vi "Test Bumpy Terrain.vi"   [LabVIEW 2017]
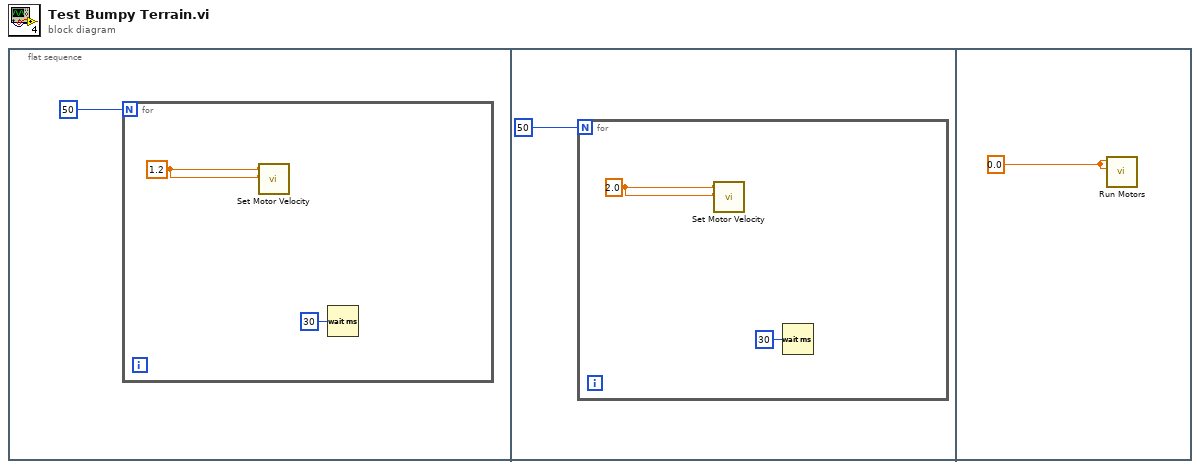
[diagram p0: block diagram]
diagram:
  n1 = flat-sequence {
    frame #0 {
      n2 = for {
        N: 50 -> [_]
        w3 = 1.2 ("Left motor speed (-1..1)")
        n3 = call "Set Motor Velocity.vi"("Right motor speed rev/s"=w3, "Left motor speed rev/s"=w3) -> ()  [unwired: 10 in]
        n4 = Wait (ms)(milliseconds to wait=u32 30) -> ()  [unwired: 1 out]
      }
    }
    frame #1 {
      n5 = for {
        N: 50 -> [_]
        w6 = 2.0 ("Left motor speed (-1..1)")
        n6 = call "Set Motor Velocity.vi"("Right motor speed rev/s"=w6, "Left motor speed rev/s"=w6) -> ()  [unwired: 10 in]
        n7 = Wait (ms)(milliseconds to wait=u32 30) -> ()  [unwired: 1 out]
      }
    }
    frame #2 {
      w7 = 0.0 ("Left motor speed (-1..1)")
      n8 = call "Run Motors.vi"("Right motor side (-1..1)"=w7, "Left motor speed (-1..1)"=w7) -> ()  [unwired: 10 in]
    }
  }
